vi "IMUcalc Bias.vi"(7 "Number of loops":i32, 10 "error in (no error)":errorcluster) -> (1 "Bias":T1, 3 "error out":errorcluster)   [LabVIEW 2016]
doc: "Inputs\nNumber of loops\n\nOutputs\nBias\n\nThis VI calculates the bias for the accelerometer and gyroscopic readings, the bias is later used when the lean angle is calculated. When this VI runs it is important that the bicycle stands still in an upright position so the IMU values are as accurate as possible."
uses:
  <vilib>/Platform/TimedLoop/XDataNode/timing_clust.ctl
  <vilib>/Platform/TimedLoop/XDataNode/nitl_modes.ctl
  <vilib>/Platform/TimedLoop/XDataNode/wakeup.ctl
  <vilib>/Platform/TimedLoop/XDataNode/XDataNode.xnode
  <vilib>/Platform/TimedLoop/XDataNode/XDNodeRunTimeDep.lvlib
panel:
  out "Z gyro bias":dbl
  out "Y gyro bias":dbl
  out "X gyro bias":dbl
  out "Z acc bias":dbl
  out "Y acc bias":dbl
  out "X acc bias":dbl
  out "Accel, Gyro":u16[](array[numeric])
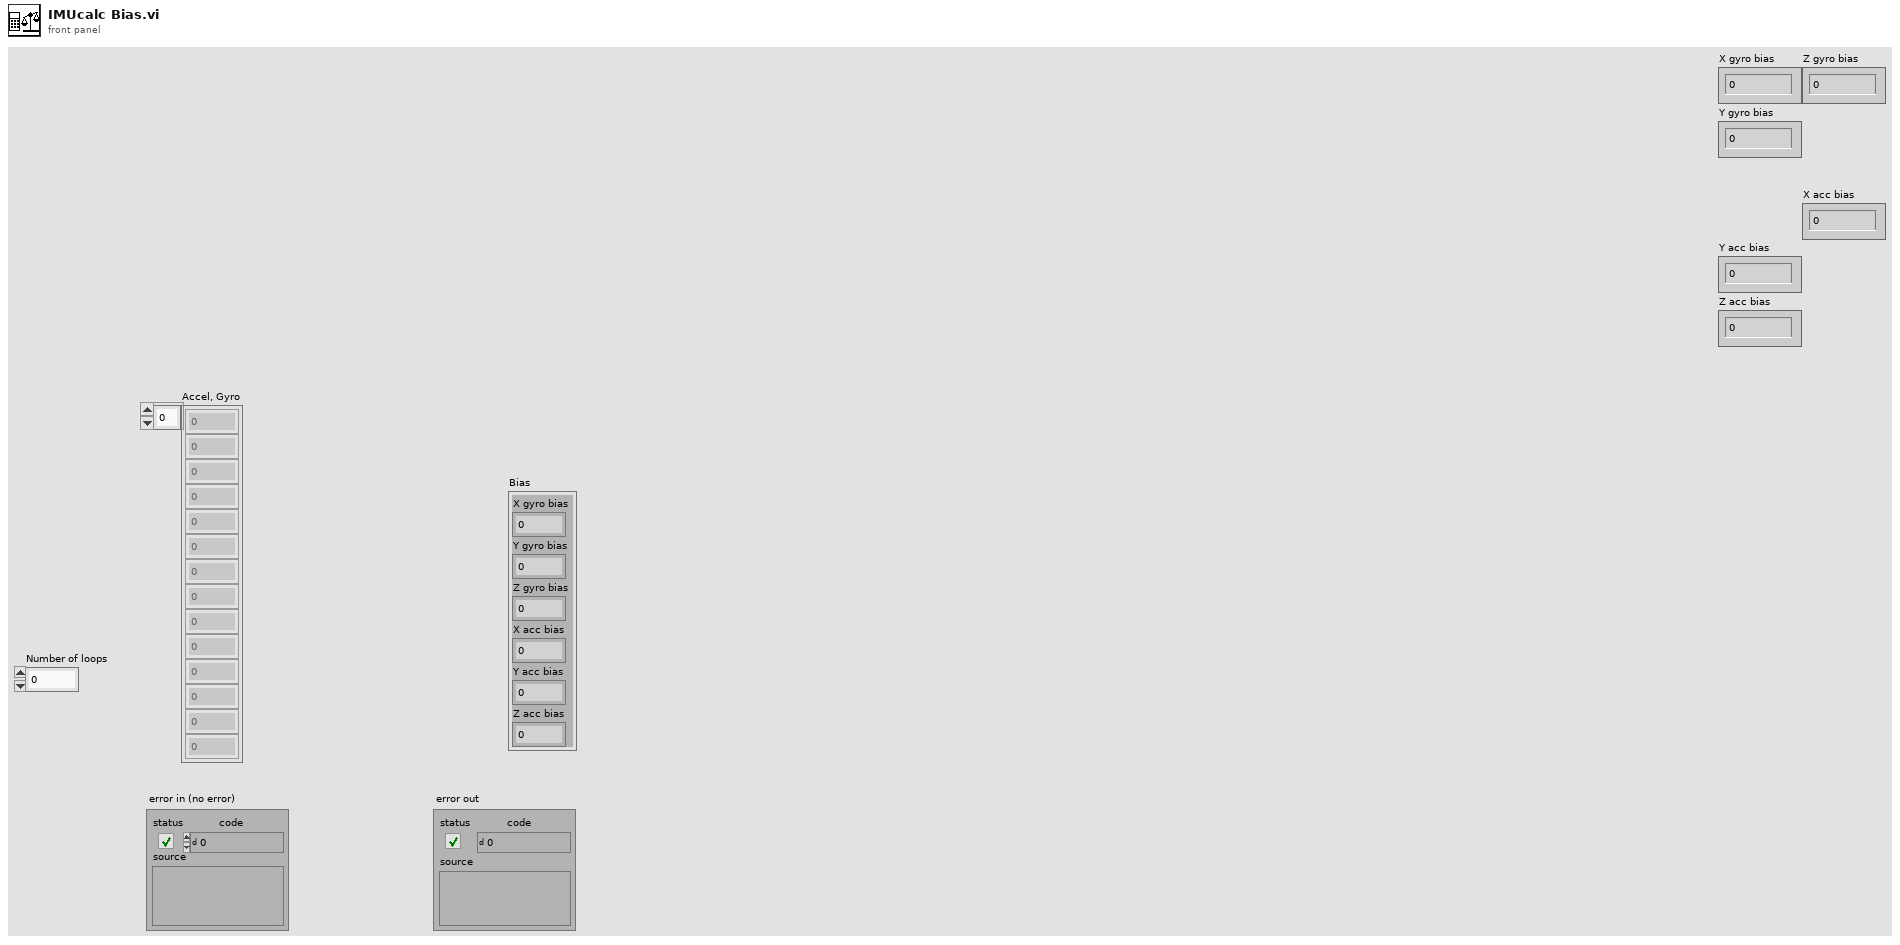
[diagram p1: front panel]
types:
  T1 = cluster{"X gyro bias":dbl, "Y gyro bias":dbl, "Z gyro bias":dbl, "X acc bias":dbl, "Y acc bias":dbl, "Z acc bias":dbl}
  T2 = typedef "XDNodeRunTimeDep.lvlib/timing_clust.ctl" = cluster{"Expected End [f-1]":u64, "Actual End [f-1]":u64, "Finished Late? [f-1]":bool, "Expected End [i-1]":u64, "Actual End [i-1]":u64, "Finished Late? [i-1]":bool, "Expected Start [i]":u64, "Actual Start [i]":u64, "Expected Start [f]":u64, "Actual Start [f]":u64, "Source Name":string, "Structure Name":string, "Period":i64, "Deadline":i64, "Offset":i64, "Start":i64, "Priority":i32, "Timeout":i32, "Mode":T3, "Wakeup Reason":T4, "Error":errorcluster, "Source Type":string, "Secondary Source Type":string, "Global End Time":u64, "Global Start Time":u64, "Frame Duration":u64, "Iteration Duration":u64, "Assigned CPU":i32, "I/O Scan Engine Mode":u32}
  T3 = typedef "XDNodeRunTimeDep.lvlib/nitl_modes.ctl" = enum32{"No Change", "Process missed periods, maintain original phase", "Discard missed periods, maintain original phase", "Process missed periods, ignore original phase", "Discard missed periods, ignore original phase"}
  T4 = typedef "XDNodeRunTimeDep.lvlib/wakeup.ctl" = enum32{"Normal", "Aborted", "Asynchronous wakeup", "Timing source error", "Timed loop error", "Timeout"}
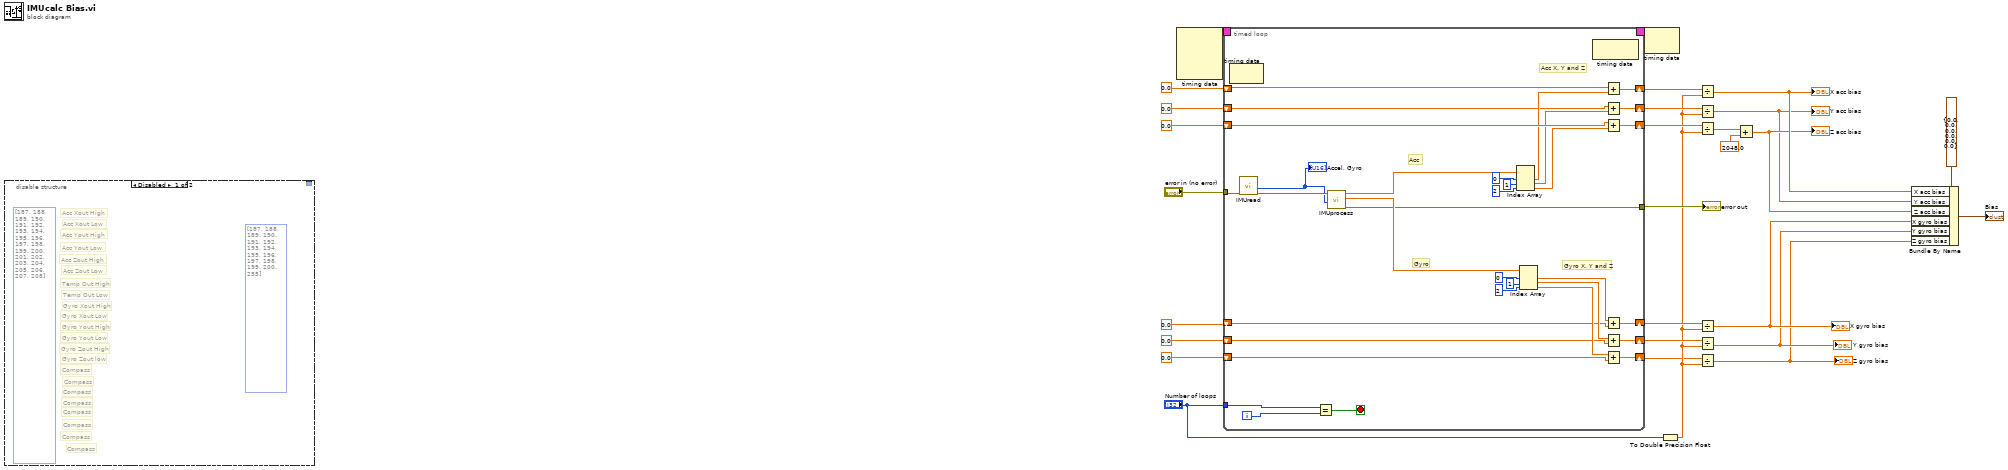
[diagram p0: block diagram]
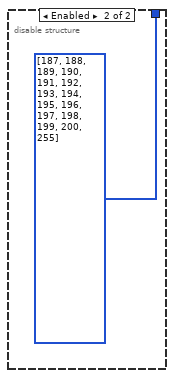
[diagram p2: hidden frame]
diagram:
  n1 = disable-structure shown="Disabled" {
    disable-tunnel: [_ u16[] [187, 188, 189, 190, 191, 192, 193, 194, 195, 196, 197, 198, 199, 200, 255] ("Frames to Write")] -> _
    frame Disabled {
      (unwired) u16[] [187, 188, 189, 190, 191, 192, 193, 194, 195, 196, 197, 198, 199, 200, 201, 202, 203, 204, 205, 206, 207, 208] ("Frames to Write")
      (unwired) u16[] [187, 188, 189, 190, 191, 192, 193, 194, 195, 196, 197, 198, 199, 200, 255] ("Frames to Write")
      # "Compass"
      # "Compass"
      # "Compass"
      # "Compass"
      # "Compass"
      # "Compass"
      # "Compass"
      # "Compass"
      # "Gyro Zout low"
      # "Gyro Zout High"
      # "Gyro Yout Low"
      # "Gyro Yout High"
      # "Gyro Xout Low"
      # "Gyro Xout High"
      # "Temp Out Low"
      # "Temp Out High"
      # "Acc Zout Low"
      # "Acc Zout High"
      # "Acc Yout Low"
      # "Acc Yout High"
      # "Acc Xout Low"
      # "Acc Xout High"
    }
    frame Enabled {
    }
  }
  n2 = node-c288() -> (w28:T2)  [unwired: 4 in]
  n3 = timed-loop {
    timing: w28 -> [_]
    timing-out: [_] -> w27
    shift-right: [w52] -> w18
    shift-left: 0.0 -> [w54]
    shift-right: [w51] -> w17
    shift-left: 0.0 -> [w48]
    shift-right: [w50] -> w16
    shift-left: 0.0 -> [w53]
    tunnel: [w45] -> w23
    tunnel: "error in (no error)" -> [w44]
    shift-right: [w43] -> w15
    shift-left: 0.0 -> [w37]
    shift-right: [w42] -> w14
    shift-left: 0.0 -> [w36]
    shift-right: [w41] -> w1
    shift-left: 0.0 -> [w35]
    tunnel: "Number of loops" -> [w31]
    i -> [w34]
    stop <- w30 stop-if-true
    # "Gyro"
    # "Acc"
    # "Gyro X, Y and Z"
    # "Acc X, Y and Z"
    n4 = node-c288() -> ()  [unwired: 1 in, 1 out]
    n5 = call "IMUread.vi"("error in (no error)"=w44) -> ("error out"=w62:errorcluster, "Accel, Gyro"=w33:u16[])  [unwired: 9 in]
    "Accel, Gyro" <- w33
    n6 = Equal?(x=w31, y=w34) -> (x = y?=w30:bool)
    n7 = call "IMUprocess.vi"("Frames Read"=w33, "error in (no error)"=w62) -> ("error out"=w45:errorcluster, "Gyro deg/s"=w59:dbl[], "Accel g's"=w32:dbl[])  [unwired: 7 in]
    n8 = Index Array(array=w32, index #1=0 ("index"), index #2=1 ("index"), index #3=2 ("index")) -> (element #1=w49:dbl, element #2=w47:dbl, element #3=w46:dbl)
    n9 = Index Array(array=w59, index #1=0 ("index"), index #2=1 ("index"), index #3=2 ("index")) -> (element #1=w40:dbl, element #2=w39:dbl, element #3=w38:dbl)
    n10 = node-c288() -> ()  [unwired: 1 in, 1 out]
    n11 = Add(x=w54, y=w49) -> (x+y=w52:dbl)
    n12 = Add(x=w48, y=w47) -> (x+y=w51:dbl)
    n13 = Add(x=w53, y=w46) -> (x+y=w50:dbl)
    n14 = Add(x=w40, y=w37) -> (x+y=w43:dbl)
    n15 = Add(x=w39, y=w36) -> (x+y=w42:dbl)
    n16 = Add(x=w38, y=w35) -> (x+y=w41:dbl)
  }
  "error out" <- w23
  n17 = node-c288(w27) -> ()  [unwired: 1 out]
  n18 = To Double Precision Float(number="Number of loops") -> (double precision float=w3:dbl)
  n19 = Divide(x=w18, y=w3) -> (x/y=w10:dbl)
  "X acc bias" <- w10
  n20 = Divide(x=w17, y=w3) -> (x/y=w5:dbl)
  "Y acc bias" <- w5
  n21 = Divide(x=w16, y=w3) -> (x/y=w8:dbl)
  n22 = Divide(x=w15, y=w3) -> (x/y=w13:dbl)
  "X gyro bias" <- w13
  n23 = Divide(x=w14, y=w3) -> (x/y=w12:dbl)
  "Y gyro bias" <- w12
  n24 = Divide(x=w1, y=w3) -> (x/y=w11:dbl)
  "Z gyro bias" <- w11
  n25 = Add(x=w8, y=2048.0) -> (x+y=w7:dbl)
  "Z acc bias" <- w7
  n26 = Bundle By Name(cluster=T1 {"X gyro bias"=0.0, "Y gyro bias"=0.0, "Z gyro bias"=0.0, "X acc bias"=0.0, "Y acc bias"=0.0, "Z acc bias"=0.0} ("Cluster"), "X acc bias"=w10, "Y acc bias"=w5, "Z acc bias"=w7, "X gyro bias"=w13, "Y gyro bias"=w12, "Z gyro bias"=w11) -> (→"Bias":T1)
